vi "USBSwitchInitFail.vi"() -> (2 "Transducer":enum16{"Transducer 1", "Transducer 2"}(ring), 3 "Abort":bool)   [LabVIEW 2022 SP3]
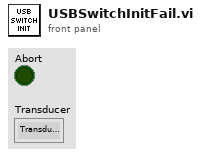
[diagram p1: front panel]
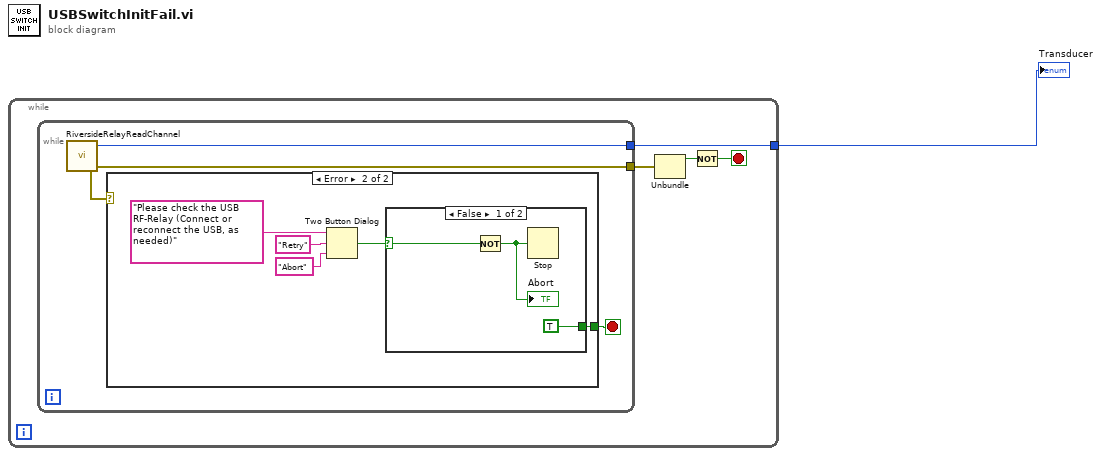
[diagram p0: block diagram]
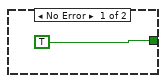
[diagram p2: hidden frame]
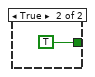
[diagram p3: hidden frame]
diagram:
  n1 = while {
    tunnel: [w5] -> w1
    stop <- w2 stop-if-true
    n2 = while {
      tunnel: [w8] -> w5
      tunnel: [w6] -> w4
      stop <- w7 stop-if-true
      n3 = call "RiversideRelayReadChannel.vi"() -> ("Transducer"=w8:enum16{"Transducer 1", "Transducer 2"}, "error out"=w6:errorcluster)  [unwired: 6 in]
      n4 = case shown="Error" w6 {
        tunnel: [TRUE ("true") w10] -> w7
        frame No Error {
        }
        frame Error {
          n5 = Two Button Dialog(message="Please check the USB RF-Relay (Connect or reconnect the USB, as needed)", 1:"Abort" ("F button name (\"Cancel\")"), 2:"Retry" ("button name (\"OK\")")) -> (T button?=w11:bool)
          n6 = case shown="False" w11 {
            selector: w11 -> [w16 _]
            tunnel: [TRUE ("true") TRUE ("true")] -> w10
            frame False {
              n7 = Not(x=w16) -> (.not. x?=w15:bool)
              "Abort" <- w15
              n8 = Stop(stop? (T)=w15) -> ()
            }
            frame True {
            }
          }
        }
      }
    }
    n9 = Unbundle(w4) -> ("status"=w3:bool)  [unwired: 2 out]
    n10 = Not(x=w3) -> (.not. x?=w2:bool)
  }
  "Transducer" <- w1
